vi "Do.vi"(8 "error in (no error)":errorcluster, 10 "Actor in":refnum<class "Actor.lvclass">, 11 "Configure Width Trigger Source [WT] Msg":refnum<class "Configure Width Trigger Source [WT] Msg.lvclass">) -> (0 "error out":errorcluster, 2 "Actor out":refnum<class "Actor.lvclass">)   [LabVIEW 2015, in "CS++Scope.lvlib" / "Configure Width Trigger Source [WT] Msg.lvclass"]
doc: "This VI delivers the message to the actor by calling the appropriate method(s) on the actor."
uses:
  Configure Width Trigger Source [WT] Msg.lvclass
  CS++Scope/CS++Scope.lvclass
  <vilib>/ActorFramework/Actor/Actor.lvclass
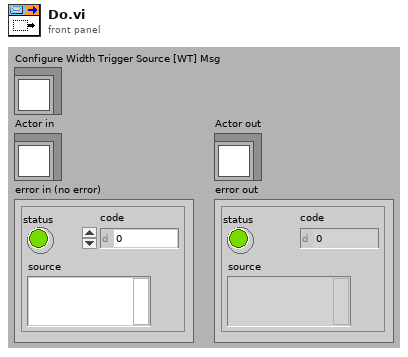
[diagram p1: front panel]
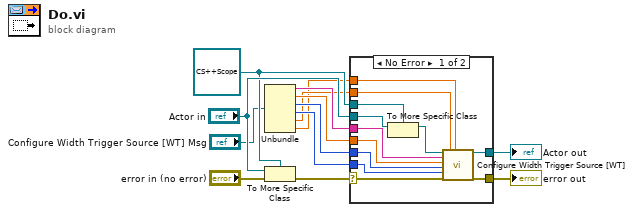
[diagram p0: block diagram]
diagram:
  w8 = refnum<class "CS++Scope.lvclass"> refnum ("Actor in")
  n1 = Unbundle ("Main-Unbundle")("Configure Width Trigger Source [WT] Msg") -> (w6:string, w5:dbl[unit], w4:i32, w3:i32, w2:dbl[unit], w1:dbl[unit])
  n2 = To More Specific Class(target class=w8, reference="Actor in", error in="error in (no error)") -> (error out=w12:errorcluster)  [unwired: 1 out]
  n3 = case shown="No Error" w12 {
    selector: w12 -> [w23 w27]
    tunnel: [w25 w27] -> w11
    tunnel: [w24 w26] -> w10
    tunnel: "Actor in" -> [w22 w26]
    tunnel: w8 -> [w21 _]
    tunnel: w6 -> [w19 _]
    tunnel: w5 -> [w18 _]
    tunnel: w4 -> [w17 _]
    tunnel: w3 -> [w16 _]
    tunnel: w2 -> [w15 _]
    tunnel: w1 -> [w14 _]
    frame No Error {
      n4 = To More Specific Class(target class=w21, reference=w22) -> (specific class reference=w20:refnum<class "CS++Scope.lvclass">)  [unwired: 1 in, 1 out]
      n5 = call-dynamic "Configure Width Trigger Source [WT].vi"("CS++Scope"=w20, "trigger source (\"CHANNEL1\")"=w19, "trigger level (0.0 V)"=w18, "width condition (Within)"=w17, "width polarity (Positive)"=w16, "error in (no error)"=w23, "width low threshold (1.0 E-9 V)"=w15, "width high threshold (2.0 E-9 V)"=w14) -> ("CS++Scope out"=w24:refnum<class "CS++Scope.lvclass">, "error out"=w25:errorcluster)  [unwired: 10 in]
    }
    frame Error {
    }
  }
  "error out" <- w11
  "Actor out" <- w10
